vi "Parallel Executing Test Code.vi"(9 "Test Complete Event":refnum<user-event>, 10 "Positions":u32[](array[numeric]), 11 "LCM1 Power On in":refnum<class "LCM1 Power On.lvclass">) -> ()   [LabVIEW 2015, in "LCM1 Power On.lvclass"]
uses:
  LCM1 Power On.lvclass
  RF Common Tests/Common RF Tests/RF Common Tests.lvclass
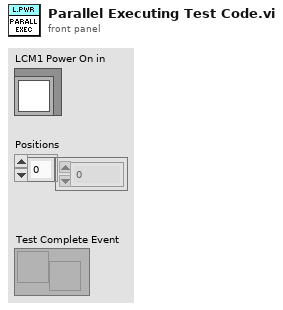
[diagram p1: front panel]
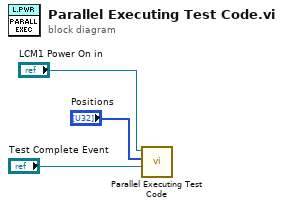
[diagram p0: block diagram]
diagram:
  n1 = call-parent "Parallel Executing Test Code.vi"("Test Complete Event"="Test Complete Event", "Positions"="Positions", "Parallel Test in"="LCM1 Power On in") -> ()  [unwired: 9 in]
